vi "processAllFrames.vi"(0 "Def Proc":refnum<class "ConfigProc.lvclass">, 1 "cropLinesOut":dbl, 3 "Output Path":path, 4 "Scan":refnum<class "Scan.lvclass">, 5 "Buffer in":dbl[][](array[numeric]), 6 "Progress":refnum<vi>, 7 "FFTW3 arrays":T3, 9 "Display":refnum<vi>, 10 "wavenumber vector":dbl[](array[numeric]), 11 "error in":errorcluster, 12 "Updated camera":T2, 14 "OCT filename out":string) -> (15 "error out":errorcluster)   [LabVIEW 2017]
uses:
  classes/SoftwareObjects/ConfigProc/ConfigProc.lvclass
  <vilib>/vision/Image Controls.llb/IMAQ Image.ctl
  classes/Scans/Scan.lvclass
  classes/Scans/Scan.lvclass/Scan.ctl
  classes/Scans/Read B scans.vi
  classes/Scans/Read Total A-scans per frame.vi
  classes/Scans/Read Total B-Scans.vi
panel:
  out "Proc time (s)":dbl
  out "size(s)":i32[](array[numeric])
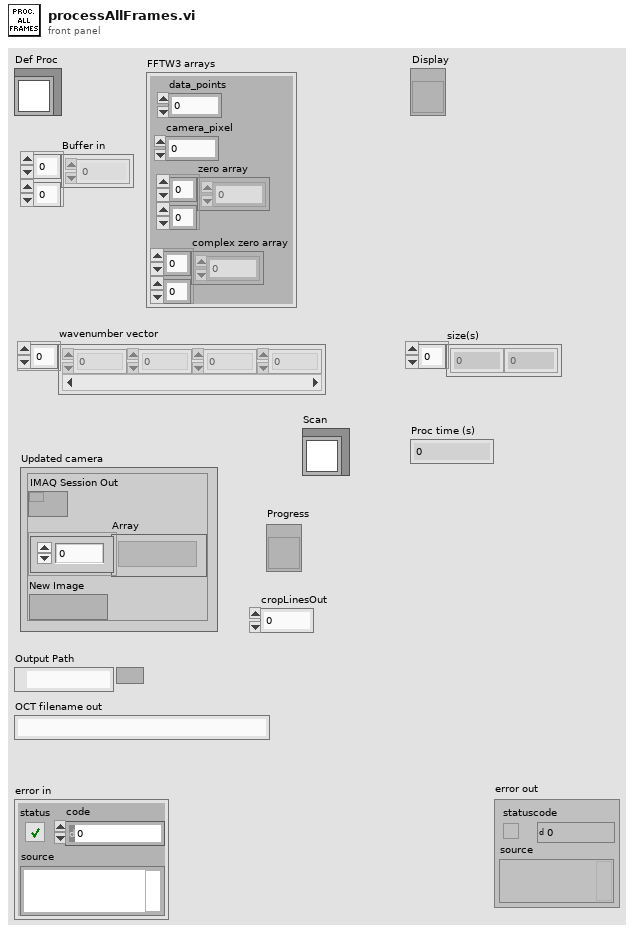
[diagram p1: front panel]
types:
  T1 = typedef "IMAQ Image.ctl" = refnum<image>
  T2 = cluster{"IMAQ Session Out":refnum<k11>, "Array":T1[], "New Image":T1}
  T3 = cluster{"data_points":i32, "camera_pixel":i32, "zero array":dbl[][], "complex zero array":dbl[][]}
  T4 = typedef "Image Type" = u32
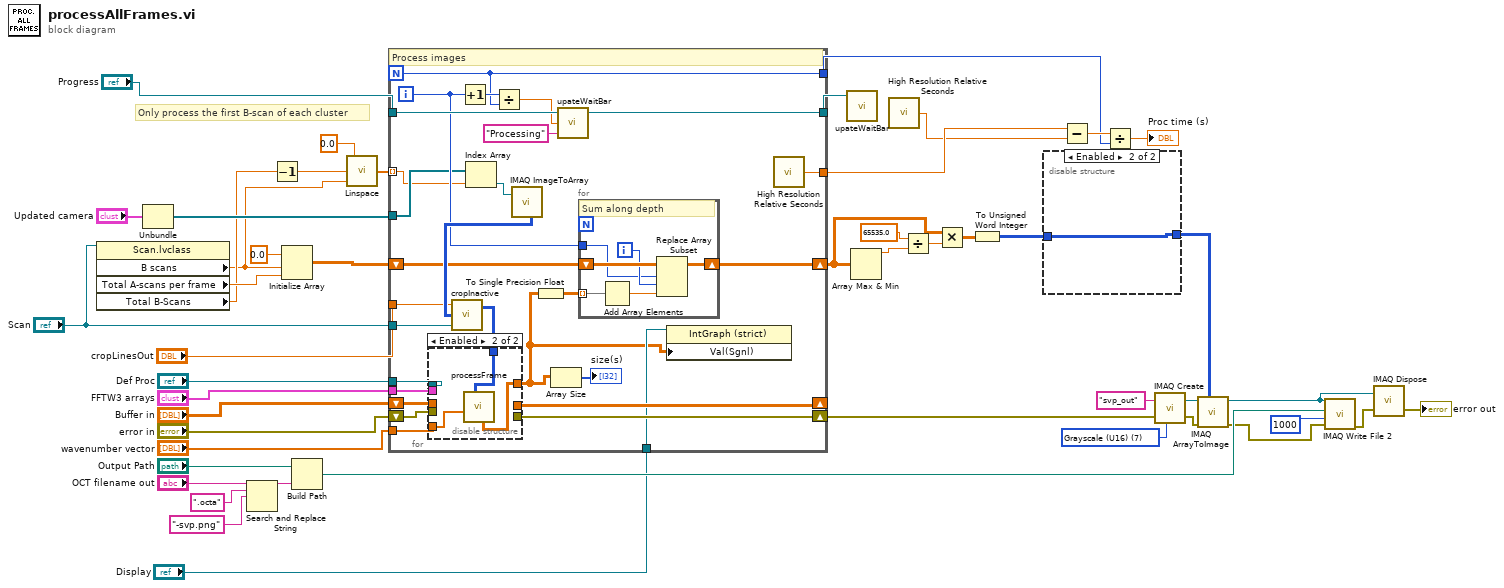
[diagram p0: block diagram]
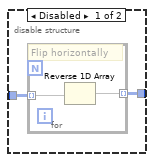
[diagram p2: hidden frame]
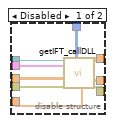
[diagram p3: hidden frame]
diagram:
  w38 = T4 7 items=["Grayscale (U8)", "Grayscale (I16)", "Grayscale (SGL)", "Complex (CSG)", "RGB (U32)", "HSL (U32)", "RGB (U64)", "Grayscale (U16)"] ("Image Type")
  # "Only process the first B-scan of each cluster"
  n1 = property class="Scan.lvclass"(reference="Scan") -> ("B scans"=w2:dbl, "Total A-scans per frame"=w31:dbl, "Total B-Scans"=w4:dbl)  [unwired: 1 in, 2 out]
  n2 = Unbundle("Updated camera") -> ("Array"=w15:T1[])  [unwired: 2 out]
  n3 = Search and Replace String(input string="OCT filename out", search string=".octa", replace string="-svp.png" ("replace string (\"\")")) -> (result string=w41:string)  [unwired: 5 in, 3 out]
  n4 = Decrement(x=w4) -> (x-1=w5:dbl)
  n5 = Initialize Array(sgl 0.0 ("element"), w2, w31) -> (w30:sgl[][])
  n6 = Build Path(base path="Output Path", name or relative path=w41) -> (appended path=w40:path)
  n7 = call "Linspace.vi"("NumElements"=w2, "End"=w5, "Start"=0.0) -> ("Array"=w1:dbl[])
  n8 = for {
    N -> [w54]
    tunnel: "Def Proc" -> [w76]
    shift-right: [w71] -> _
    shift-left: "Buffer in" -> [w74]
    tunnel: "wavenumber vector" -> [w73]
    shift-right: [w72] -> w20
    shift-left: "error in" -> [w75]
    tunnel: "FFTW3 arrays" -> [w70]
    tunnel: w15 -> [w51]
    tunnel: "Scan" -> [w67]
    shift-right: [w65] -> w24
    shift-left: w30 -> [w66]
    tunnel: "Progress" -> [w62]
    tunnel: [w57] -> w13
    tunnel: "cropLinesOut" -> [w56]
    tunnel: [w55] -> w11
    tunnel: [w54] -> w8
    tunnel: "Display" -> [w53]
    tunnel: w1 -> [w50] mode=indexing
    i -> [w61]
    # "Process images"
    n9 = Increment(x=w61) -> (x+1=w60:i32)
    n10 = Index Array(array=w51, index=w50) -> (element=w49:T1)
    n11 = Divide(x=w60, y=w54) -> (x/y=w59:dbl)
    n12 = call "IMAQ ImageToArray"("Image"=w49) -> ("Image Pixels (U16)"=w69:u16[][])  [unwired: 3 in, 4 out]
    n13 = call "cropInactive.vi"("Scan in"=w67, "Whole camera frame"=w69, "cropLines"=w56) -> ("Cropped camera frame"=w68:u16[][])  [unwired: 1 in]
    n14 = disable-structure shown="Enabled" {
      disable-tunnel: w76 -> [w85 _]
      disable-tunnel: w75 -> [w84 _]
      disable-tunnel: w74 -> [w83 _]
      disable-tunnel: w73 -> [w82 w86]
      disable-tunnel: [w81 _] -> w72
      disable-tunnel: [w80 _] -> w71
      disable-tunnel: w70 -> [w79 _]
      disable-tunnel: w68 -> [w78 w88]
      disable-tunnel: [w77 w87] -> w52
      frame Disabled {
        n15 = call "getIFT_callDLL.vi"("Processing Configuration"=w85, "FFTW3 arrays"=w79, "Buffer in"=w83, "error in (no error)"=w84, "Interferogram"=w78, "Spectrum calibration"=w82) -> ("Depth Profile"=w77:dbl[][], "Buffer out"=w80:dbl[][], "error in (no error) 2"=w81:errorcluster)  [unwired: 10 in, 1 out]
      }
      frame Enabled {
        n16 = call "processFrame.vi"("Image"=w88, "wavenumber vector"=w86) -> ("Image out"=w87:dbl[][])  [unwired: 9 in]
      }
    }
    n17 = To Single Precision Float(number=w52) -> (single precision float=w64:sgl[][])
    n18 = Array Size(array=w52) -> (size(s)=→"size(s)":i32[])
    n19 = call "upateWaitBar.vi"("waitbar text"="Processing", "waitbar value [0,1]"=w59, "Progress"=w62) -> ("Updated Progress"=w57:refnum<vi>)  [unwired: 2 in]
    n20 = for {
      tunnel: w64 -> [w91] mode=indexing
      shift-right: [w94] -> w65
      shift-left: w66 -> [w93]
      tunnel: w61 -> [w90]
      i -> [w92]
      # "Sum along depth"
      n21 = Add Array Elements(numeric array=w91) -> (sum=w89:sgl)
      n22 = Replace Array Subset(array=w93, new element=w89, index (row)=w90, index (col)=w92) -> (w94:sgl[][])
    }
    n23 = property class="IntGraph (strict)"(reference=w53, "Val(Sgnl)"=w52) -> ()  [unwired: 1 in, 2 out]
    n24 = call <vilib>:"High Resolution Relative Seconds.vi"() -> ("relative seconds"=w55:dbl)
  }
  n25 = call "upateWaitBar.vi"("Progress"=w13) -> ()  [unwired: 4 in, 1 out]
  n26 = Array Max & Min(array=w24) -> (max value=w25:sgl)  [unwired: 3 out]
  n27 = call <vilib>:"High Resolution Relative Seconds.vi"() -> ("relative seconds"=w10:dbl)
  n28 = Divide(x=sgl 65535.0, y=w25) -> (x/y=w28:sgl)
  n29 = Multiply(x=w24, y=w28) -> (x*y=w27:sgl[][])
  n30 = To Unsigned Word Integer(number=w27) -> (unsigned 16bit integer=w26:u16[][])
  n31 = disable-structure shown="Enabled" {
    disable-tunnel: w26 -> [w96 w99]
    disable-tunnel: [w95 w99] -> w21
    frame Disabled {
      n32 = for {
        tunnel: w96 -> [w98] mode=indexing
        tunnel: [w97] -> w95 mode=indexing
        # "Flip horizontally"
        n33 = Reverse 1D Array(array=w98) -> (reversed array=w97:u16[])
      }
    }
    frame Enabled {
    }
  }
  n34 = Subtract(x=w11, y=w10) -> (x-y=w9:dbl)
  n35 = Divide(x=w9, y=w8) -> (x/y=→"Proc time (s)":dbl)
  n36 = call "IMAQ Create"("Image Name"="svp_out", "Image Type"=w38, "error in (no error)"=w20) -> ("New Image"=w37:T1, "error out"=w19:errorcluster)  [unwired: 2 in]
  n37 = call "IMAQ ArrayToImage"("Image Pixels (U16)"=w21, "error in (no error)"=w19, "Image"=w37) -> ("error out"=w18:errorcluster, "Image Out"=w35:T1)  [unwired: 7 in]
  n38 = call-poly "IMAQ Write File 2"("error in (no error)"=w18, "Image Quality"=u32 1000, "File Path"=w40, "Image"=w35) -> ("error out"=w34:errorcluster)  [unwired: 6 in, 1 out]
  n39 = call "IMAQ Dispose"("Image"=w35, "error in (no error)"=w34) -> ("error out"=→"error out":errorcluster)  [unwired: 4 in]
